vi "Close Waveform Stream Specification.vi"(8 "error in (no error)":errorcluster, 11 "WaveformStreamSpecification":T1) -> (0 "error out":errorcluster)   [LabVIEW 2020, in "NI_VS Waveform Streaming Interface.lvlib"]
doc: "Closes a waveform stream specification you opened with the New Waveform Stream Specification VI."
uses:
  <vilib>/NI VeriStand/Execution/WaveformStreaming/NI_VS Waveform Streaming Interface.lvlib
  <vilib>/NI VeriStand/Execution/WaveformStreaming/WaveformStreamSpecification.ctl
  NationalInstruments.VeriStand.ClientAPI
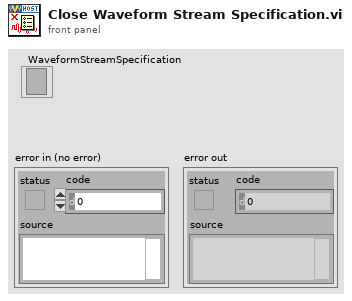
[diagram p1: front panel]
types:
  T1 = typedef "NI_VS Waveform Streaming Interface.lvlib/WaveformStreamSpecification.ctl" = refnum<k24>
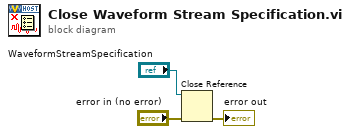
[diagram p0: block diagram]
diagram:
  n1 = Close Reference(reference="WaveformStreamSpecification", error in (no error)="error in (no error)") -> (error out=→"error out":errorcluster)
